vi "GenerateArray.vi"(9 "Stop":dbl=8.0 format="%#_13g", 10 "Start":dbl=1.0 format="%#_13g", 11 "Array_size":i32) -> (3 "Array":u8[](array[numeric]))   [LabVIEW 2015]
panel:
  out "min value":u8
  out "max value":u8
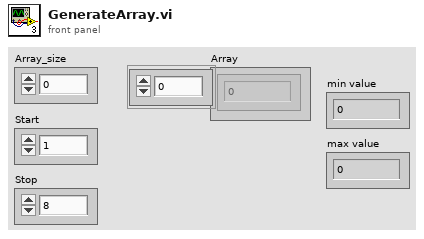
[diagram p1: front panel]
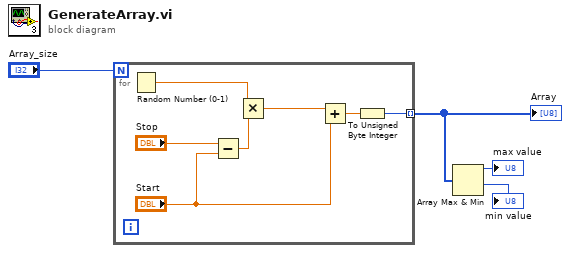
[diagram p0: block diagram]
diagram:
  n1 = for {
    N: "Array_size" -> [_]
    tunnel: [w8] -> w3 mode=indexing
    n2 = Random Number (0-1)() -> (number: 0 to 1=w11:dbl)
    n3 = Subtract(x="Stop", y="Start") -> (x-y=w5:dbl)
    n4 = Multiply(x=w11, y=w5) -> (x*y=w10:dbl)
    n5 = Add(x=w10, y="Start") -> (x+y=w9:dbl)
    n6 = To Unsigned Byte Integer(number=w9) -> (unsigned 8bit integer=w8:u8)
  }
  "Array" <- w3
  n7 = Array Max & Min(array=w3) -> (max value=→"max value":u8, min value=→"min value":u8)  [unwired: 2 out]
